vi "Doc Dir.vi"(8 "error in (no error)":errorcluster) -> (0 "error out":errorcluster, 3 "appended path":path)   [LabVIEW 2014, in "lvprj2html.lvlib"]
uses:
  lvprj2html.lvlib
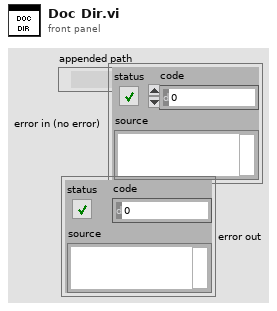
[diagram p1: front panel]
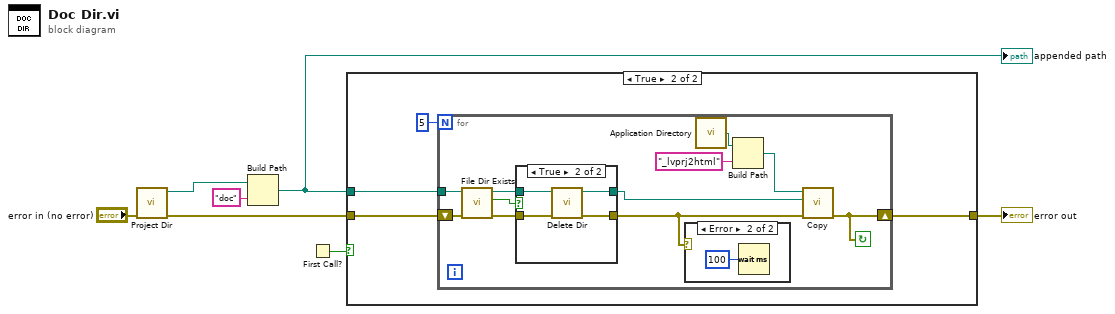
[diagram p0: block diagram]
diagram:
  n1 = call "Project Dir.vi"("error in (no error)"="error in (no error)") -> ("error out"=w3:errorcluster, "path"=w5:path)  [unwired: 9 in]
  n2 = Build Path(base path=w5, name or relative path="doc") -> (appended path=w6:path)
  "appended path" <- w6
  n3 = First Call?() -> (First Call?: T/F=w7:bool)
  n4 = case shown="True" w7 {
    tunnel: w6 -> [_ w10]
    tunnel: w3 -> [w8 w11]
    tunnel: [w8 w12] -> w1
    frame False {
    }
    frame True {
      n5 = for {
        N: 5 -> [_]
        tunnel: w10 -> [w16]
        shift-right: [w14] -> w12
        shift-left: w11 -> [w17]
        stop <- w14 continue-if-true
        n6 = call "File Dir Exists.vi"("error in (no error)"=w17, "path"=w16) -> ("error out"=w18:errorcluster, "exists"=w19:bool, "path out"=w15:path)  [unwired: 7 in]
        n7 = case shown="True" w19 {
          tunnel: w15 -> [w26 w30]
          tunnel: [w26 w27] -> w20
          tunnel: w18 -> [w25 w29]
          tunnel: [w25 w28] -> w13
          frame False {
          }
          frame True {
            n8 = call "Delete Dir.vi"("error in (no error)"=w29, "dup path"=w30) -> ("error out"=w28:errorcluster, "deleted path"=w27:path)  [unwired: 8 in]
          }
        }
        n9 = case shown="Error" w13 {
          frame No Error {
          }
          frame Error {
            n10 = Wait (ms)(milliseconds to wait=u32 100) -> ()  [unwired: 1 out]
          }
        }
        n11 = call <vilib>:"Application Directory.vi"() -> ("Application Directory"=w22:path)
        n12 = Build Path(base path=w22, name or relative path="_lvprj2html") -> (appended path=w21:path)
        n13 = call "Copy.vi"("error in (no error)"=w13, "dst"=w20, "src"=w21) -> ("error out"=w14:errorcluster)  [unwired: 8 in]
      }
    }
  }
  "error out" <- w1
